vi "I2C_end.vi"(8 "Time SCL Low":u32, 11 "Time SCL High":u32) -> ()   [LabVIEW 2019]
uses:
  <vilib>/rvi/eio/common/nirviEmuTemplateMethod_errors.vi
  <vilib>/eio/EIONode/EIONode.xnode
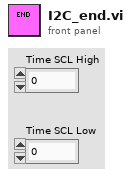
[diagram p1: front panel]
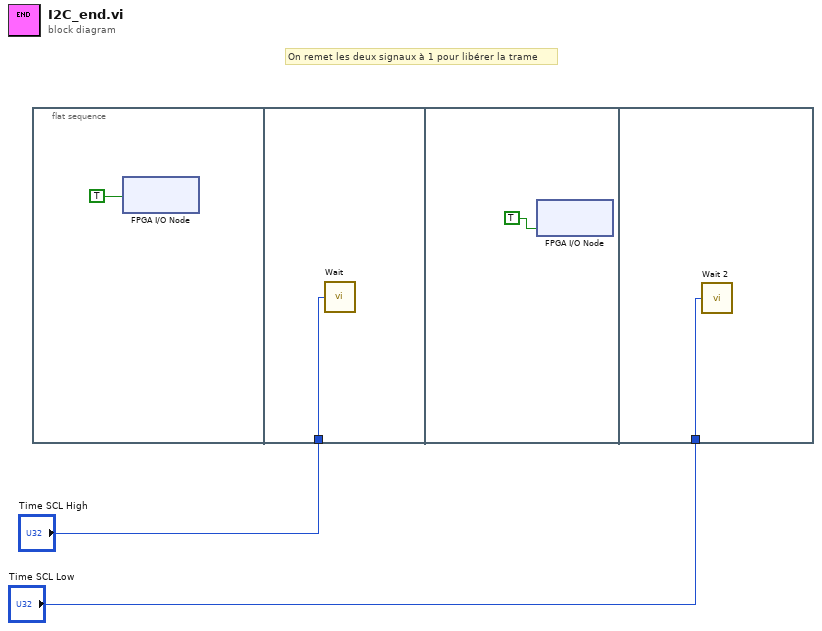
[diagram p0: block diagram]
diagram:
  # "On remet les deux signaux à 1 pour libérer la trame"
  n1 = flat-sequence {
    tunnel: "Time SCL High" -> [w4]
    tunnel: "Time SCL Low" -> [w6]
    frame #0 {
      n2 = xnode "FPGA I/O Node"("SCL"=TRUE ("Digital Out")) -> ()  [unwired: 1 in, 1 out]
    }
    frame #1 {
      n3 = call "Wait"("Count(uSec)"=w4) -> ()  [unwired: 1 out]
    }
    frame #2 {
      n4 = xnode "FPGA I/O Node"("SDA"=TRUE ("Digital Out")) -> ()  [unwired: 1 in, 1 out]
    }
    frame #3 {
      n5 = call "Wait 2"("Count(uSec)"=w6) -> ()  [unwired: 1 out]
    }
  }
